vi "TCP&IP_Client_Test.vi"() -> ()   [LabVIEW 2017]
panel:
  in  "Exit":bool
  out "数据输出":string
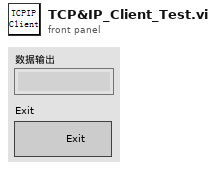
[diagram p1: front panel]
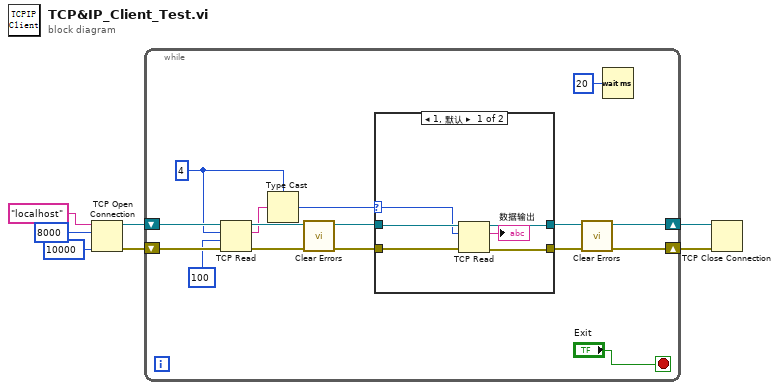
[diagram p0: block diagram]
diagram:
  n1 = TCP Open Connection(address="localhost" ("地址"), remote port or service name=u16 8000 ("远程端口或服务名称"), timeout ms (60000)=10000 ("超时毫秒(60000)")) -> (connection ID=w4:refnum<k5>, error out=w5:errorcluster)  [unwired: 2 in]
  n2 = while {
    shift-right: [w8] -> w2
    shift-left: w5 -> [w21]
    shift-right: [w15] -> w3
    shift-left: w4 -> [w20]
    stop <- "Exit" stop-if-true
    w17 = 4 ("读取的字节")
    n3 = TCP Read(connection ID=w20, bytes to read=w17, error in (no error)=w21, 9:100 ("超时毫秒(25000)")) -> (connection ID out=w19:refnum<k5>, data out=w18:string, error out=w14:errorcluster)  [unwired: 1 in]
    n4 = Type Cast(type=w17, x=w18) -> (*(type *) &x=w16:i32)
    n5 = call <vilib>:"Clear Errors.vi"("error in (no error)"=w14) -> ("error out"=w9:errorcluster)  [unwired: 5 in, 1 out]
    n6 = case shown="1, 默认" w16 {
      selector: w16 -> [w23 _]
      tunnel: w19 -> [w27 w29]
      tunnel: [w25 w29] -> w15
      tunnel: w9 -> [w26 w28]
      tunnel: [w24 w28] -> w13
      frame 1, Default {
        n7 = TCP Read(connection ID=w27, bytes to read=w23, error in (no error)=w26) -> (connection ID out=w25:refnum<k5>, data out=→"数据输出":string, error out=w24:errorcluster)  [unwired: 2 in]
      }
      frame ..0 {
      }
    }
    n8 = call <vilib>:"Clear Errors.vi"("error in (no error)"=w13) -> ("error out"=w8:errorcluster)  [unwired: 5 in, 1 out]
    n9 = Wait (ms)(milliseconds to wait=u32 20 ("等待时间（毫秒）")) -> ()  [unwired: 1 out]
  }
  n10 = TCP Close Connection(connection ID=w3, error in (no error)=w2) -> ()  [unwired: 1 in, 2 out]
